vi "HH coil setup - BK9129B_devOBD.VI"(6 "Arduino VISA in":refnum<visa-resource-name>="Arduino", 8 "setup enabled?":bool=TRUE, 9 "number":i32=2, 10 "VISA resource name":refnum<visa-resource-name>="BK9123A_moe", 11 "coil polarity":bool) -> (1 "Z current out (mA)":dbl=800.0, 2 "Y current out (mA)":dbl=1200.0, 3 "X current out (mA)":dbl=30.0)   [LabVIEW 2018]
panel:
  in  "Table Control":string[][](table)=[["Field (G)", "X curr pos (mA)", "X curr neg (mA)", "Y curr pos (mA)", "Y curr neg (mA)", "Z curr pos (mA)", "Z curr neg (mA)"], ["9", "-20", "20", "-1500", "1500", "-975", "975"], ["14", "-30", "30", "-2250", "2250", "-1462.5", "1462.5"]]
  in  "Serial Configuration":T1={"Parity(0:none)"=0, "Baud Rate (9600)"=9600, "Data Bits(8)"=8, "Flow Control(None)"=0, " Stop Bits(1.0)"=10} {"Stop Bits(1.0)" items=["1.0"=10, "1.5"=15, "2.0"=20]; "Flow Control(None)" items=["None", "XON/XOFF", "RTS/CTS", "XON/XOFF & RTS/CTS", "DTR/DSR", "XON/XOFF & DTR/DSR"]; "Data Bits(8)" items=["7"=7, "8"=8]; "Baud Rate (9600)" items=["2400"=2400, "4800"=4800, "9600"=9600, "19200"=19200, "38400"=38400]; "Parity(0:none)" items=["None", "Odd", "Even", "Mark", "Space"]}
  in  "Z voltage max (V)":dbl=15.0
  in  "Y voltage max (V)":dbl=15.0
  in  "X voltage max (V)":dbl=5.0
  out "pin states 2-13":bool[](array[boolean])=[FALSE, FALSE, FALSE, TRUE, TRUE, TRUE, FALSE, FALSE, FALSE, FALSE, FALSE, FALSE]
  # "update Nov 21 2018\nuse current signs to set polarity"
  # "5"
  # "12"
  # "current polarity\noff = negative\non = positive"
  # "5-7=TTL\n12=LED"
  # "for BK9129B\ncoil 1 is for Z\ncoil 2 is for Y\ncoil 3 is for X (the weak one)"
  # "for arduino\npin 5 is for Z\npin 6 is for Y\npin 7 is for X (the weak one)\n\nusually do them all together though"
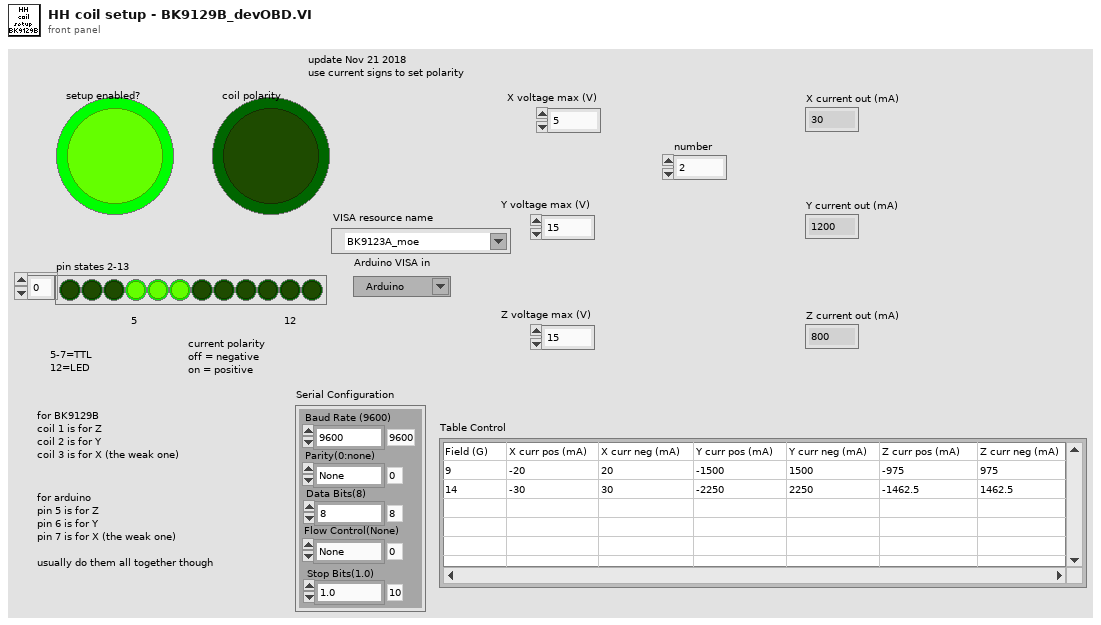
[diagram p1: front panel]
types:
  T1 = cluster{"Parity(0:none)":u16, "Baud Rate (9600)":u16, "Data Bits(8)":u16, "Flow Control(None)":u16, " Stop Bits(1.0)":u16}
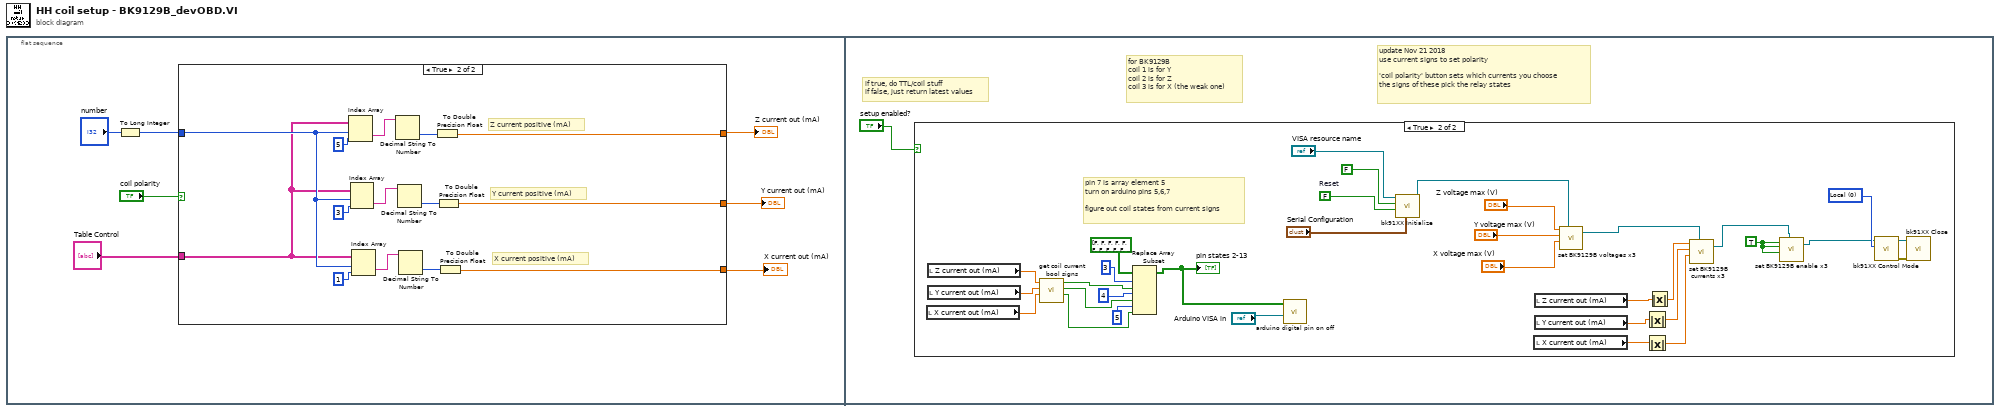
[diagram p0: block diagram]
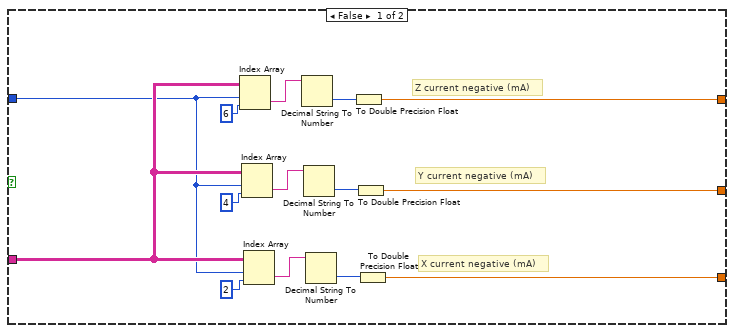
[diagram p2: hidden frame]
diagram:
  n1 = flat-sequence {
    frame #0 {
      n2 = To Long Integer(number="number") -> (32bit integer=w2:i32)
      n3 = case shown="True" "coil polarity" {
        tunnel: [w8 w25] -> w6
        tunnel: [w9 w24] -> w5
        tunnel: [w10 w23] -> w4
        tunnel: w2 -> [w11 w29]
        tunnel: "Table Control" -> [w12 w22]
        frame False {
          # "Z current negative (mA)"
          # "Y current negative (mA)"
          # "X current negative (mA)"
          n4 = Index Array(array=w12, index (row)=w11, index (col)=6 ("disabled index (col)")) -> (element=w20:string)
          n5 = Index Array(array=w12, index (row)=w11, index (col)=4 ("disabled index (col)")) -> (element=w19:string)
          n6 = Index Array(array=w12, index (row)=w11, index (col)=2 ("disabled index (col)")) -> (element=w17:string)
          n7 = Decimal String To Number(string=w20) -> (number=w21:i32)  [unwired: 2 in, 1 out]
          n8 = Decimal String To Number(string=w19) -> (number=w18:i32)  [unwired: 2 in, 1 out]
          n9 = Decimal String To Number(string=w17) -> (number=w16:i32)  [unwired: 2 in, 1 out]
          n10 = To Double Precision Float(number=w21) -> (double precision float=w8:dbl)
          n11 = To Double Precision Float(number=w18) -> (double precision float=w9:dbl)
          n12 = To Double Precision Float(number=w16) -> (double precision float=w10:dbl)
        }
        frame True {
          # "X current positive (mA)"
          # "Y current positive (mA)"
          # "Z current positive (mA)"
          n13 = Index Array(array=w22, index (row)=w29, index (col)=5 ("disabled index (col)")) -> (element=w34:string)
          n14 = Index Array(array=w22, index (row)=w29, index (col)=3 ("disabled index (col)")) -> (element=w33:string)
          n15 = Index Array(array=w22, index (row)=w29, index (col)=1 ("disabled index (col)")) -> (element=w31:string)
          n16 = Decimal String To Number(string=w34) -> (number=w35:i32)  [unwired: 2 in, 1 out]
          n17 = Decimal String To Number(string=w33) -> (number=w32:i32)  [unwired: 2 in, 1 out]
          n18 = Decimal String To Number(string=w31) -> (number=w30:i32)  [unwired: 2 in, 1 out]
          n19 = To Double Precision Float(number=w35) -> (double precision float=w25:dbl)
          n20 = To Double Precision Float(number=w32) -> (double precision float=w24:dbl)
          n21 = To Double Precision Float(number=w30) -> (double precision float=w23:dbl)
        }
      }
      "X current out (mA)" <- w4
      "Y current out (mA)" <- w5
      "Z current out (mA)" <- w6
    }
    frame #1 {
      # "update Nov 21 2018\nuse current signs to set polarity\n\n'coil polarity' button sets which currents you choose\nthe signs of these pick the relay states"
      # "for BK9129B\ncoil 1 is for Y\ncoil 2 is for Z\ncoil 3 is for X (the weak one)"
      # "if true, do TTL/coil stuff\nif false, just return latest values"
      n22 = case shown="True" "setup enabled?" {
        frame False {
        }
        frame True {
          w53 = u16 0 items=["Local", "Remote"] ("Control Mode(1:Remote)")
          w55 = TRUE
          w64 = FALSE items=["OFF", "ON", "OFF", "ON"]  # Reset
          # "pin 7 is array element 5\nturn on arduino pins 5,6,7\n\nfigure out coil states from current signs"
          n23 = local read "X current out (mA)"() -> (w47:dbl)
          n24 = local read "Z current out (mA)"() -> (w45:dbl)
          n25 = local read "Y current out (mA)"() -> (w46:dbl)
          n26 = call "get coil current bool signs.vi"("X current (mA)"=w47, "Y current (mA)"=w46, "Z current (mA)"=w45) -> ("x sign"=w48:bool, "y sign"=w49:bool, "z sign"=w50:bool)  [unwired: 6 in]
          n27 = Replace Array Subset(array=bool[] [FALSE, FALSE, FALSE, FALSE, FALSE, FALSE, FALSE, FALSE, FALSE, FALSE, FALSE, FALSE] ("pin states 2-13 2"), new element #1=w50, index #1=3 ("index"), new element #2=w49, index #2=4 ("index"), new element #3=w48, index #3=5 ("index")) -> (w38:bool[])
          "pin states 2-13" <- w38
          n28 = call "arduino digital pin on off.vi"("Arduino VISA in"="Arduino VISA in", "pin states 2-13"=w38) -> ()  [unwired: 10 in]
          n29 = call "bk91XX Initialize.vi"("Serial Configuration"="Serial Configuration", "Reset (True)"=w64, "ID Query (True)"=FALSE, "VISA resource name"="VISA resource name") -> ("VISA resource name out"=w58:refnum<visa-resource-name>)  [unwired: 6 in, 1 out]
          n30 = local read "X current out (mA)"() -> (w42:dbl)
          n31 = local read "Z current out (mA)"() -> (w43:dbl)
          n32 = local read "Y current out (mA)"() -> (w44:dbl)
          n33 = call "set BK9129B voltages x3.vi"("voltage in 1 (V)"="Z voltage max (V)", "voltage in 2 (V)"="Y voltage max (V)", "voltage in 3 (V)"="X voltage max (V)", "VISA in"=w58) -> ("VISA out"=w57:refnum<visa-resource-name>)  [unwired: 1 in, 1 out]
          n34 = Absolute Value(x=w44) -> (abs(x)=w40:dbl)
          n35 = Absolute Value(x=w42) -> (abs(x)=w41:dbl)
          n36 = Absolute Value(x=w43) -> (abs(x)=w39:dbl)
          n37 = call "set BK9129B currents x3.vi"("current in 1 (mA)"=w39, "current in 2 (mA)"=w40, "current in 3 (mA)"=w41, "VISA in"=w57) -> ("VISA out"=w56:refnum<visa-resource-name>)  [unwired: 1 in, 1 out]
          n38 = call "set BK9129B enable x3.vi"("ch 1 state"=w55, "ch 2 state"=w55, "ch 3 state"=w55, "VISA in"=w56) -> ("VISA out"=w51:refnum<visa-resource-name>)  [unwired: 1 in, 1 out]
          n39 = call "bk91XX Control Mode.vi"("Control Mode (1: Remote)"=w53, "VISA resource name"=w51) -> ("error out"=w52:errorcluster, "VISA resource name out"=w54:refnum<visa-resource-name>)  [unwired: 8 in]
          n40 = call "bk91XX Close.vi"("error in (no error)"=w52, "VISA resource name"=w54) -> ()  [unwired: 9 in, 1 out]
        }
      }
    }
  }
